vi "Open_File_for_write.vi"(8 "advisory dialog? (display:T)":bool=TRUE, 9 "append to file? (new file:F)":bool, 11 "file path":path) -> (0 "error out":errorcluster, 3 "refnum":refnum<file>)   [LabVIEW 2014]
doc: "Opens an existing file, creates a new file, or replaces an existing file, programmatically or interactively using dialog. You can optionally specify a dialog prompt, default file name, start path, or filter pattern, and you can specify open and deny modes when opening a file, plus group and permission when creating a new file. Use this VI with the intermediate Write File+ or Read File+ VIs described below.\n\nfile path is the path name of the file. If file path is empty (default value) or is Not A Path, the VI displays a File dialog box from which you can select a file. Error 43 occurs if the user cancels the dialog. \n\nfunction is the operation to perform:\n\n 0 (open) opens an existing file. Error 7 occurs if the file cannot be found.\n \n 1 (open or create) opens an existing file or creates a new file if one does not exist.\n\n 2 (create or replace) creates a new file or replaces a file if it exists and you give permission. Replacement is done by opening the file and setting EOF to 0. Error 43 occurs if the user elects to disallow the replacement using dialog. \n\n 3 (create) creates a new file. Error 8 occurs if the file already exists.\n\nadvisory dialog? Set TRUE (default) if you want a dialog if function=0 and the file does not exist, or if function=2 or 3 and the file exists.\n\nprompt is the message that appears below the list of files and directories in the file dialog.\n\ndefault name is the initial file name that appears in the selection box of the file dialog.\n\nstart path is the path name to the initially displayed directory in a file dialog. The default value is Not A Path, which is the path to the last directory shown in a file dialog.\n\npattern is the match pattern specification to display only certain types of files or directories. See the description of the File Dialog function for more information.\n\nerror in is a cluster of three elements (error?, code, and source) that describe the upstream error state, that is, the existance of any error preceeding the execution of the VI. The VI executes normally only if no incoming error exists; otherwise it merely passes the error in value to error out. error? is TRUE if an error occurred; the default value is FALSE. code is the error code; the default value is 0. source is in most cases the name of the VI or function that produced the error; the default value is an empty string.\n\nnew file path is the path of the file opened or created. You can use this output to determine the path of a file that you open or create using dialog. new file path returns Not A Path if the user selects Cancel from the dialog box.\n\nrefnum is the reference number of the open file. The value is Not A Refnum if the file cannot be opened.\n\nfile size is the size of the file in bytes; it is also the location of the end of file.\n\nerror out is a cluster of three elements (error?, code, and source) that describe the error state following the execution of the VI. If an incoming error does not exist, the VI executes normally and error out describes the VI's error state; if an incoming error exists, error out equals error in."
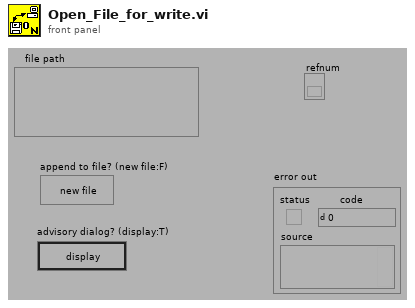
[diagram p1: front panel]
types:
  T1 = enum16{"deny read/write", "deny write-only", "deny none"}
  T2 = enum16{"open", "replace", "create", "open or create", "replace or create", "replace or create with confirmation"}
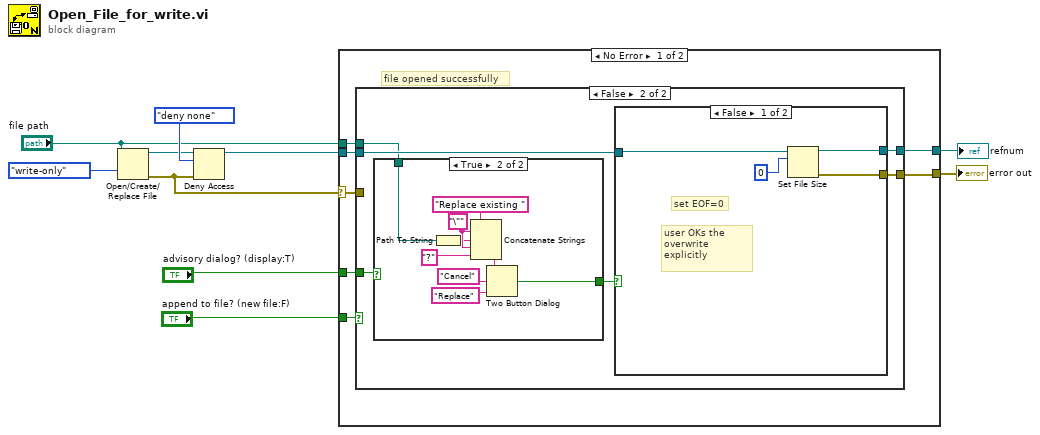
[diagram p0: block diagram]
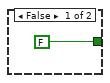
[diagram p3: hidden frame]
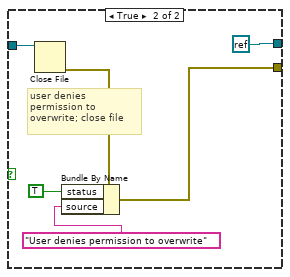
[diagram p4: hidden frame]
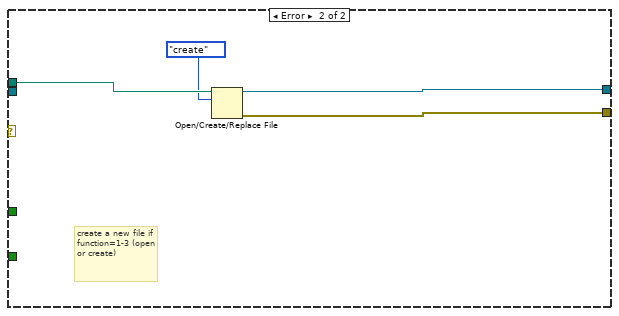
[diagram p5: hidden frame]
diagram:
  n1 = Open/Create/Replace File(file path (use dialog)="file path", access (0:read/write)=enum16{"read/write", "read-only", "write-only"}."write-only") -> (refnum out=w4:refnum<file>, error out=w1:errorcluster)  [unwired: 1 in, 4 out]
  n2 = Deny Access(4:w1, 6:T1."deny none" ("deny mode (2)"), 7:w4) -> (3:w9:refnum<file>)  [unwired: 1 out]
  n3 = case shown="No Error" w1 {
    selector: w1 -> [w11 _]
    tunnel: "file path" -> [w17 w47]
    tunnel: "append to file? (new file:F)" -> [w12 _]
    tunnel: [w16 w49] -> w8
    tunnel: w9 -> [w15 _]
    tunnel: "advisory dialog? (display:T)" -> [w14 _]
    tunnel: [w13 w48] -> w6
    frame No Error {
      # "file opened successfully"
      n4 = case shown="False" w12 {
        tunnel: w17 -> [_ w20]
        tunnel: [w19 w25] -> w16
        tunnel: w15 -> [w19 w24]
        tunnel: w14 -> [_ w22]
        tunnel: [w18 w21] -> w13
        tunnel: w11 -> [w18 _]
        frame True {
          # "file is now open; proceed if function=1 (open or create)"
        }
        frame False {
          n5 = case shown="True" w22 {
            tunnel: [FALSE w34] -> w23
            tunnel: w20 -> [_ w27]
            frame False {
            }
            frame True {
              w29 = "\""
              n6 = Path To String(path=w27) -> (string=w28:string)
              n7 = Concatenate Strings("Replace existing ", w29, w28, w29, "?") -> (w35:string)
              n8 = Two Button Dialog(message=w35, 1:"Replace", 2:"Cancel") -> (T button?=w34:bool)
            }
          }
          n9 = case shown="False" w23 {
            tunnel: [w39 refnum<k0> refnum] -> w25
            tunnel: w24 -> [w37 w45]
            tunnel: [w38 w41] -> w21
            frame False {
              # "user OKs the overwrite explicitly"
              # "set EOF=0"
              n10 = Set File Size(6:i64 0 ("size (in bytes)"), 7:w37) -> (0:w38:errorcluster, 3:w39:refnum<file>)  [unwired: 1 in]
            }
            frame True {
              # "user denies permission to overwrite; close file"
              n11 = Close File(refnum=w45) -> (error out=w44:errorcluster)  [unwired: 1 in, 1 out]
              n12 = Bundle By Name(cluster=w44, "status"=TRUE, "source"="User denies permission to overwrite") -> (w41:errorcluster)
            }
          }
        }
      }
    }
    frame Error {
      # "create a new file if function=1-3 (open or create)"
      n13 = Open/Create/Replace File(file path (use dialog)=w47, operation (0:open)=T2."create") -> (refnum out=w49:refnum<file>, error out=w48:errorcluster)  [unwired: 1 in, 4 out]
    }
  }
  "refnum" <- w8
  "error out" <- w6
